vi "Configure Event Search (Edge).vi"(8 "error in (no error)":errorcluster, 9 "Edge Slope (0: Negative)":i32(ring) items=["Negative", "Positive", "Either"], 10 "Source Channel (0: Channel 1)":i32(ring) items=["Channel 1", "Channel 2", "Channel 3", "Channel 4"], 11 "VISA resource name":refnum<visa-resource-name>) -> (0 "error out":errorcluster, 3 "VISA resource name out":refnum<visa-resource-name>)   [LabVIEW 2023, in "Keysight-DSQx3014T.lvlib"]
doc: "Configures the event search of Edge."
uses:
  Keysight-DSQx3014T.lvlib
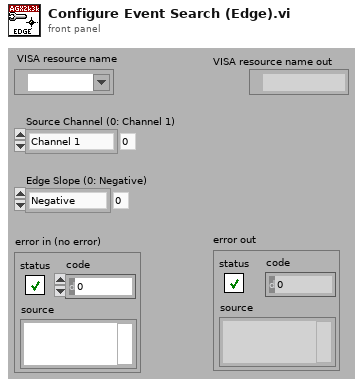
[diagram p1: front panel]
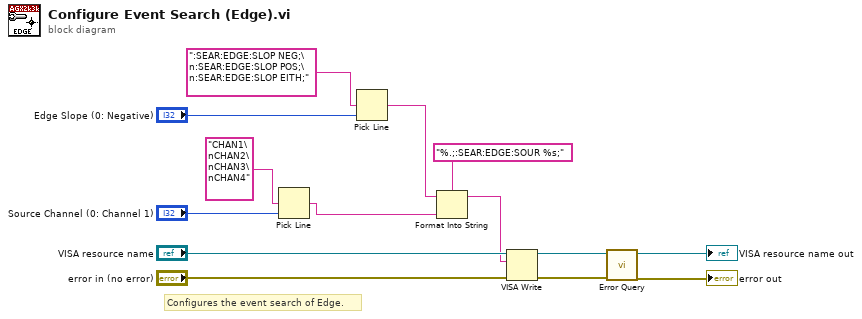
[diagram p0: block diagram]
diagram:
  # "Configures the event search of Edge."
  n1 = Pick Line(multi-line string="CHAN1\nCHAN2\nCHAN3\nCHAN4", line index="Source Channel (0: Channel 1)") -> (output string=w1:string)  [unwired: 1 out]
  n2 = Pick Line(multi-line string=":SEAR:EDGE:SLOP NEG;\n:SEAR:EDGE:SLOP POS;\n:SEAR:EDGE:SLOP EITH;", line index="Edge Slope (0: Negative)") -> (output string=w6:string)  [unwired: 1 out]
  n3 = Format Into String(format string="%.;:SEAR:EDGE:SOUR %s;", initial string=w6, w1) -> (resulting string=w5:string)  [unwired: 1 in, 1 out]
  n4 = VISA Write(VISA resource name="VISA resource name", write buffer=w5, error in (no error)="error in (no error)") -> (VISA resource name out=w10:refnum<visa-resource-name>, error out=w9:errorcluster)  [unwired: 1 out]
  n5 = call "Error Query.vi"("error in (no error)"=w9, "VISA resource name"=w10) -> ("error out"=→"error out":errorcluster, "VISA resource name out"=→"VISA resource name out":refnum<visa-resource-name>)  [unwired: 8 out]
